vi "压力位移插值.vi"(3 "压力数组":dbl[](array[numeric]), 4 "监控点位移":dbl, 5 "位移数组":dbl[](array[numeric])) -> (1 "监控点压力":dbl)   [LabVIEW 2013]
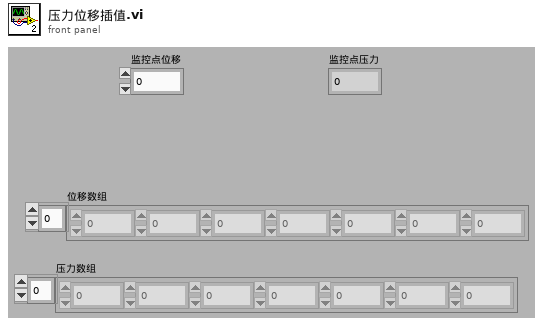
[diagram p1: front panel]
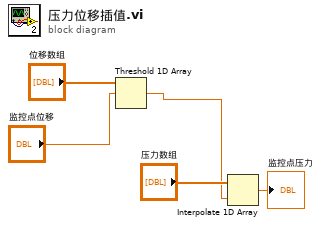
[diagram p0: block diagram]
diagram:
  n1 = Threshold 1D Array(2:"监控点位移", 3:"位移数组") -> (0:w2:dbl)  [unwired: 1 in]
  n2 = Interpolate 1D Array(1:w2, 2:"压力数组") -> (0:→"监控点压力":dbl)
